vi "4_DIOTests.vi"() -> ()   [LabVIEW 2012]
panel:
  out "BotSpeak":string="SET DIO[13],1\nGET DIO[13]\nSET PWM[0],100\nSET var,1\nSET DIO[0],1\nSET DIO[2],var\nSET DIO[var],var\nSET DIO[30],1\nSCRIPT\nSET DIO[0],1\nSET paren0,5\nSUB paren0,3\nSET tmp0,2\nMUL tmp0,paren0\nSET sum,tmp0\nSET tmp1,1\nSUB tmp1,4\nADD sum,tmp1\nSET DIO[13],sum\nSET more,DIO[0\nSET X,DIO[var]]\nend\nENDSCRIPT\nRUN&WAIT 0\nGET sum\nGET more\nGET X\n\n"
  out "expected response":string="1\r\nT\n100\r\n1\r\n1\r\n1\r\n1\r\n1\r\nstart script\r\nend script\r\n.............\nDone\r\n1\r\n1\r\n1\r\n"
  out "response":string="1\r\nT\n100\r\n1\r\n1\r\n1\r\n1\r\n1\r\nstart script\r\nend script\r\n.............\nDone\r\n1\r\n1\r\n1\r\n"
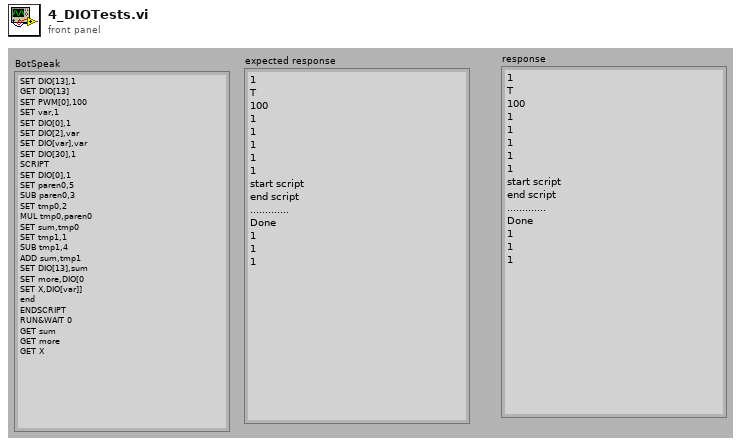
[diagram p1: front panel]
types:
  T1 = typedef "BotSpeak_Control.ctl" = cluster{"Address":string, "Reply EOF":string, "Hardware":path, "Retries":i8, "Timeout":i32}
  T2 = typedef "URAPI_Control.ctl" = cluster{"Script":string, "Whiles":u8[], "Ifs":u8[], "Supress Err":bool, "Errors":string}
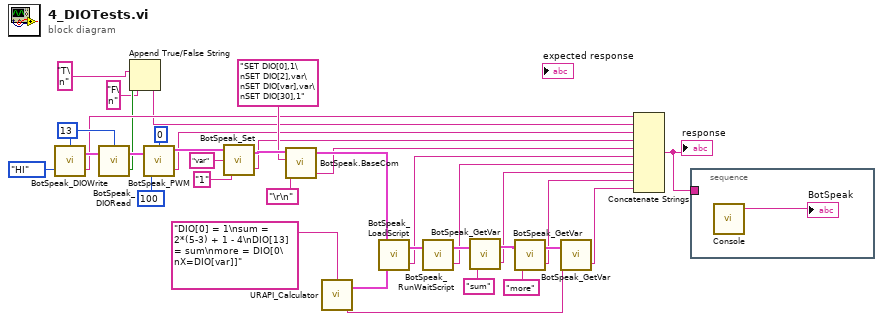
[diagram p0: block diagram]
diagram:
  w12 = u32 13 ("DIO Line")
  n1 = call <userlib>:"BotSpeak_DIOWrite.vi"("State"=enum32{"LO", "HI"}."HI", "DIO Line"=w12) -> ("response"=w7:string, "Bot Settings"=w13:T1)  [unwired: 1 in]
  n2 = call <userlib>:"BotSpeak_DIORead.vi"("Bot Settings"=w13, "DIO Line"=w12) -> ("State"=w6:bool, "Bot Settings out"=w11:T1)  [unwired: 1 in]
  n3 = Append True/False String(1:w6, 2:"F\n" ("false string"), 3:"T\n" ("true string")) -> (0:w4:string)  [unwired: 1 in]
  n4 = call <userlib>:"BotSpeak_PWM.vi"("Strength (100)"=u8 100, "Bot Settings"=w11, "PWM Line"=u8 0) -> ("response"=w5:string, "Bot Settings out"=w8:T1)
  n5 = call <userlib>:"BotSpeak_Set.vi"("value"="1", "Variable In"="var", "Bot Settings"=w8) -> ("response"=w21:string, "Bot Settings"=w33:T1)
  n6 = call <userlib>:"BotSpeak.BaseCom.vi"("Termination"="\r\n", "command"="SET DIO[0],1\nSET DIO[2],var\nSET DIO[var],var\nSET DIO[30],1" ("String"), "Bot Settings in"=w33) -> ("response"=w20:string, "Bot Settings out"=w29:T1)  [unwired: 2 in]
  n7 = call <userlib>:"URAPI_Calculator.vi"("Formula"="DIO[0] = 1\nsum = 2*(5-3) + 1 - 4\nDIO[13] = sum\nmore = DIO[0\nX=DIO[var]]") -> ("Variable Out"=w22:string, "URAPI Script"=w30:T2)  [unwired: 3 in]
  n8 = call <userlib>:"BotSpeak_LoadScript.vi"("URAPI Script"=w30, "Bot Settings"=w29) -> ("total response"=w19:string, "Bot Settings"=w28:T1)
  n9 = call <userlib>:"BotSpeak_RunWaitScript.vi"("Bot Settings"=w28) -> ("response"=w18:string, "Bot Settings"=w27:T1)  [unwired: 1 in]
  n10 = call <userlib>:"BotSpeak_GetVar.vi"("Variable In"="sum", "Bot Settings"=w27) -> ("value"=w17:string, "Bot Settings out"=w24:T1)
  n11 = call <userlib>:"BotSpeak_GetVar.vi"("Variable In"="more", "Bot Settings"=w24) -> ("value"=w16:string, "Bot Settings out"=w23:T1)
  n12 = call <userlib>:"BotSpeak_GetVar.vi"("Variable In"=w22, "Bot Settings"=w23) -> ("value"=w15:string)  [unwired: 1 out]
  n13 = Concatenate Strings(w7, w4, w5, w21, w20, w19, w18, w17, w16, w15) -> (w1:string)
  "response" <- w1
  n14 = stacked-sequence {
    tunnel: w1 -> [_]
    frame #0 {
      n15 = call <userlib>:"Console.vi"() -> ("BotSpeak"=→"BotSpeak":string)  [unwired: 4 in, 1 out]
    }
  }
